vi "Read tcp connection.vi"(8 "error in (no error)":errorcluster, 11 "IP Data Unit in":refnum<class "SMSD ADU.lvclass">) -> (0 "error out":errorcluster, 2 "tcp connection":refnum<k5>, 3 "IP Data Unit out":refnum<class "SMSD ADU.lvclass">)   [LabVIEW 2021, in "SMSD ADU.lvclass"]
uses:
  SMSD ADU.lvclass
  SMSD ADU.lvclass/SMSD ADU.ctl
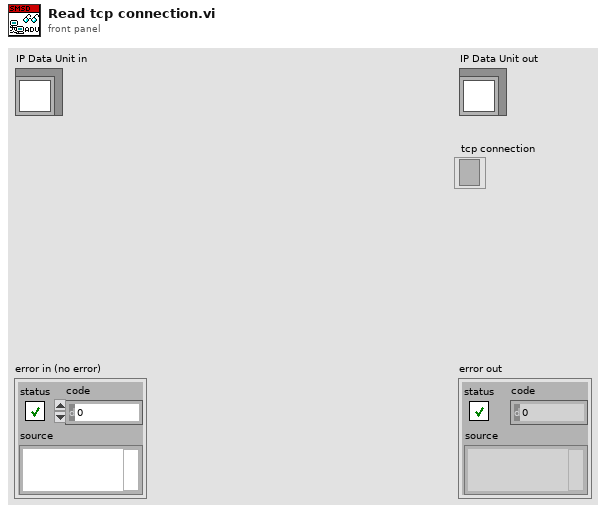
[diagram p1: front panel]
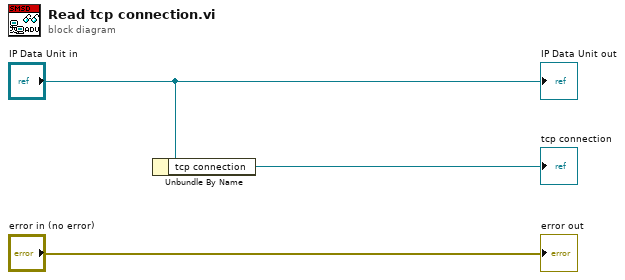
[diagram p0: block diagram]
diagram:
  n1 = Unbundle By Name("IP Data Unit in") -> ("tcp connection"=→"tcp connection":refnum<k5>)
  "error out" <- "error in (no error)"
  "IP Data Unit out" <- "IP Data Unit in"
